vi "SortFromLeft.vi"(2 "Data2":dbl[](array[numeric]), 3 "Data1":dbl[](array[numeric])) -> (0 "Second":dbl[](array[numeric]), 1 "First":dbl[](array[numeric]))   [LabVIEW 2016]
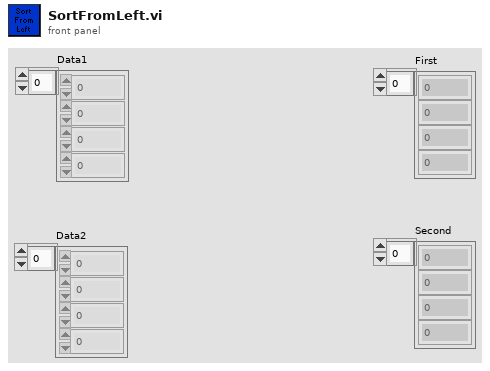
[diagram p1: front panel]
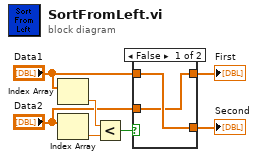
[diagram p0: block diagram]
diagram:
  n1 = Index Array(array="Data1") -> (element=w7:dbl)  [unwired: 1 in]
  n2 = Index Array(array="Data2") -> (element=w6:dbl)  [unwired: 1 in]
  n3 = Less?(x=w7, y=w6) -> (x < y?=w5:bool)
  n4 = case shown="False" w5 {
    tunnel: "Data1" -> [w9 w11]
    tunnel: [w8 w11] -> w3
    tunnel: "Data2" -> [w8 w10]
    tunnel: [w9 w10] -> w1
    frame False {
    }
    frame True {
    }
  }
  "Second" <- w1
  "First" <- w3
